vi "13.Evd.5_Ask.3.vi"() -> ()   [LabVIEW 2025]
panel:
  out "Average":bool
  out "Multiplication":bool
  out "Addition":bool
  in  "Number \nOperations":dbl
  out "Result":dbl
  in  "D":dbl
  in  "C":dbl
  in  "B":dbl
  in  "A":dbl
  out "Message":string
  in  "stop":bool
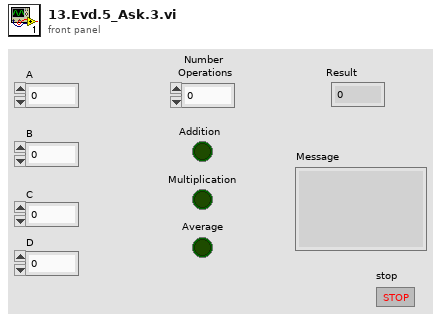
[diagram p1: front panel]
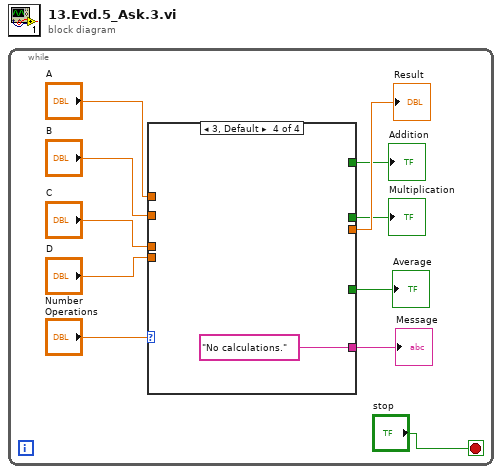
[diagram p0: block diagram]
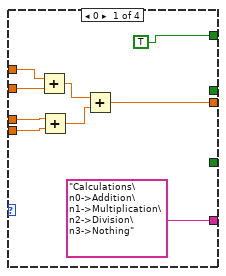
[diagram p2: hidden frame]
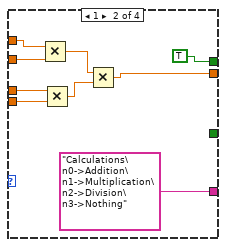
[diagram p3: hidden frame]
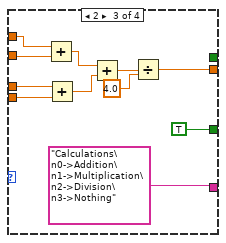
[diagram p4: hidden frame]
diagram:
  n1 = while {
    stop <- "stop" stop-if-true
    n2 = case shown="3, Default" "Number \nOperations" {
      tunnel: ["Calculations\n0->Addition\n1->Multiplication\n2->Division\n3->Nothing" "Calculations\n0->Addition\n1->Multiplication\n2->Division\n3->Nothing" "Calculations\n0->Addition\n1->Multiplication\n2->Division\n3->Nothing" "No calculations."] -> w9
      tunnel: "A" -> [w20 w29 w37 _]
      tunnel: "B" -> [w19 w28 w38 _]
      tunnel: "C" -> [w18 w24 w36 _]
      tunnel: "D" -> [w17 w23 w35 _]
      tunnel: [w14 w25 w32 _] -> w4
      tunnel: [TRUE _ _ _] -> w3
      tunnel: [_ TRUE _ _] -> w2
      tunnel: [_ _ TRUE _] -> w1
      frame 0 {
        n3 = Add(x=w20, y=w19) -> (x+y=w16:dbl)
        n4 = Add(x=w18, y=w17) -> (x+y=w15:dbl)
        n5 = Add(x=w16, y=w15) -> (x+y=w14:dbl)
      }
      frame 1 {
        n6 = Multiply(x=w29, y=w28) -> (x*y=w27:dbl)
        n7 = Multiply(x=w24, y=w23) -> (x*y=w26:dbl)
        n8 = Multiply(x=w27, y=w26) -> (x*y=w25:dbl)
      }
      frame 2 {
        n9 = Add(x=w37, y=w38) -> (x+y=w40:dbl)
        n10 = Add(x=w36, y=w35) -> (x+y=w39:dbl)
        n11 = Add(x=w40, y=w39) -> (x+y=w34:dbl)
        n12 = Divide(x=w34, y=4.0) -> (x/y=w32:dbl)
      }
      frame 3, Default {
      }
    }
    "Message" <- w9
    "Result" <- w4
    "Addition" <- w3
    "Multiplication" <- w2
    "Average" <- w1
  }
